vi "close_popup.vi"(0 "path":path, 11 "error in (no error)":errorcluster) -> (15 "error out":errorcluster)   [LabVIEW 2023]
doc: "Close the vi from given vi path"
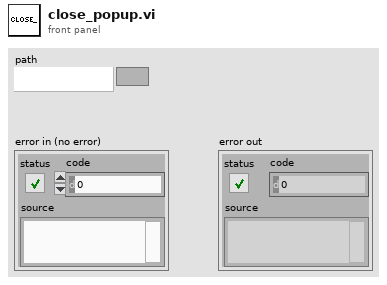
[diagram p1: front panel]
types:
  T1 = enum32{"Bad", "Idle", "Run top level", "Running"}
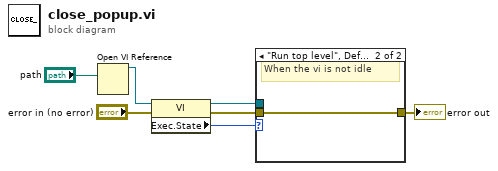
[diagram p0: block diagram]
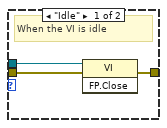
[diagram p2: hidden frame]
diagram:
  n1 = Open VI Reference(vi path="path") -> (vi reference=w4:refnum<vi>)  [unwired: 5 in, 1 out]
  n2 = property class="VI"(reference=w4, error in="error in (no error)") -> (reference out=w6:refnum<vi>, error out=w7:errorcluster, "Exec.State"=w5:T1)
  n3 = case shown="\"Run top level\", Default" w5 {
    tunnel: w6 -> [w10 _]
    tunnel: w7 -> [w9 w11]
    tunnel: [w8 w11] -> w2
    frame "Idle" {
      # "When the VI is idle"
      n4 = invoke class="VI" method="FP.Close"(reference=w10, error in=w9) -> (error out=w8:errorcluster)  [unwired: 1 in, 2 out]
    }
    frame "Run top level", Default {
      # "When the vi is not idle"
    }
  }
  "error out" <- w2
